vi "PH_Beckhoff_PP_Control.panel.vi"(0 "object ref":refnum<vi>, 5 "error in (no error)":errorcluster) -> (19 "error out":errorcluster)   [LabVIEW 2014, in "PH_Beckhoff_PP_Control.lvlib"]
doc: "This a GUI.\n\nLicense Agreement for this software:\n\nCopyright (C)\nGesellschaft für Schwerionenforschung, GSI\nPlanckstr. 1\n64291 Darmstadt\nGermany\n\nContact: D.Beck@gsi.de \n\nThis program is free software; you can redistribute it and/or modify it under the terms of the GNU General Public License as published by the Free Software Foundation; either version 2 of the license, or (at your option) any later version.\n\nThis program is distributed in the hope that it will be useful, but WITHOUT ANYW ARRANTY; without even the implied warranty of MERCHANTABILITY or FITNESS FOR A PARTICULAR PURPOSE. See the GNU General License for more details (http://www.gnu.org).\n\nGesellschaft für Schwerionenforschung, GSI\nPlanckstr. 1, 64291 Darmstadt, Germany\nFor all questions and ideas contact: M.Richter@gsi.de, H.Brand@gsi.de or D.Beck@gsi.de.\nLast update: 18-DEC-2002"
uses:
  PH_Beckhoff_PP_Control.lvlib
  PH_StatusHandler/PH_StatusHandler.GUI element.ctl
  PH_Beckhoff/PH_Beckhoff.Connectivity.ctl
  PH_Beckhoff/PH_Beckhoff.ADS Error.ctl
  PH_Beckhoff/PH_Beckhoff.Values.ctl
  PH_Beckhoff/PH_Beckhoff.Sonderklemmen Inputs.ctl
  PH_Beckhoff/PH_Beckhoff.Analog Inputs.ctl
  PH_Beckhoff/PH_Beckhoff.Scaling Type.ctl
  PH_Beckhoff/PH_Beckhoff.Analog Outputs.ctl
  PH_Beckhoff/PH_Beckhoff.Digital Inputs.ctl
  PH_Beckhoff/PH_Beckhoff.Digital Outputs.ctl
  PH_Beckhoff/PH_Beckhoff.GUI Refs.ctl
  CSCore/CSObj/CSObj.lvlib
  PH_Common/PH_Common.lvlib
  PH_Beckhoff/PH_Beckhoff.lvlib
  CSCore/CSSystem/CSSystemLib/CSSystemLib.lvlib
  PH_Class/PH_Class.lvlib
  PH_StatusHandler/PH_StatusHandler.lvlib
panel:
  in  "Tab Control":T1(tab)=enum."Mercury / Conductivity Control"
  out "Current Values":T2
  out "IP":string
  out "Connection":T9
  out "Prdc Int [ms]":i32
  out "ADS Error":T10
  out "configured?":bool
  in  "Show Info":bool
  out "Conductivity PSDB Status":u32(colorbox)=6618880 caption="PSDB"
  out "Mercury PSDB Status":u32(colorbox)=6618880 caption="PSDB"
  out "PP Conductivity Control":T12={"_Status"=0, "Device on"=16860, "Conductivity ok"=16860, "Temperature ok"=16860, "Alarm"=16860}
  out "PP Mercury Control":T13={"PHELIX Status"=0, "Device on"=16860, "Alarm"=16860, "on since:"="no info available", "Concentration"=0.0} caption="_Trigger 2 ..." {"Concentration" format="%#_7f"}
  in  "Delete":bool
  in  "Exit":bool
  # "PCS"
  # "3.40"
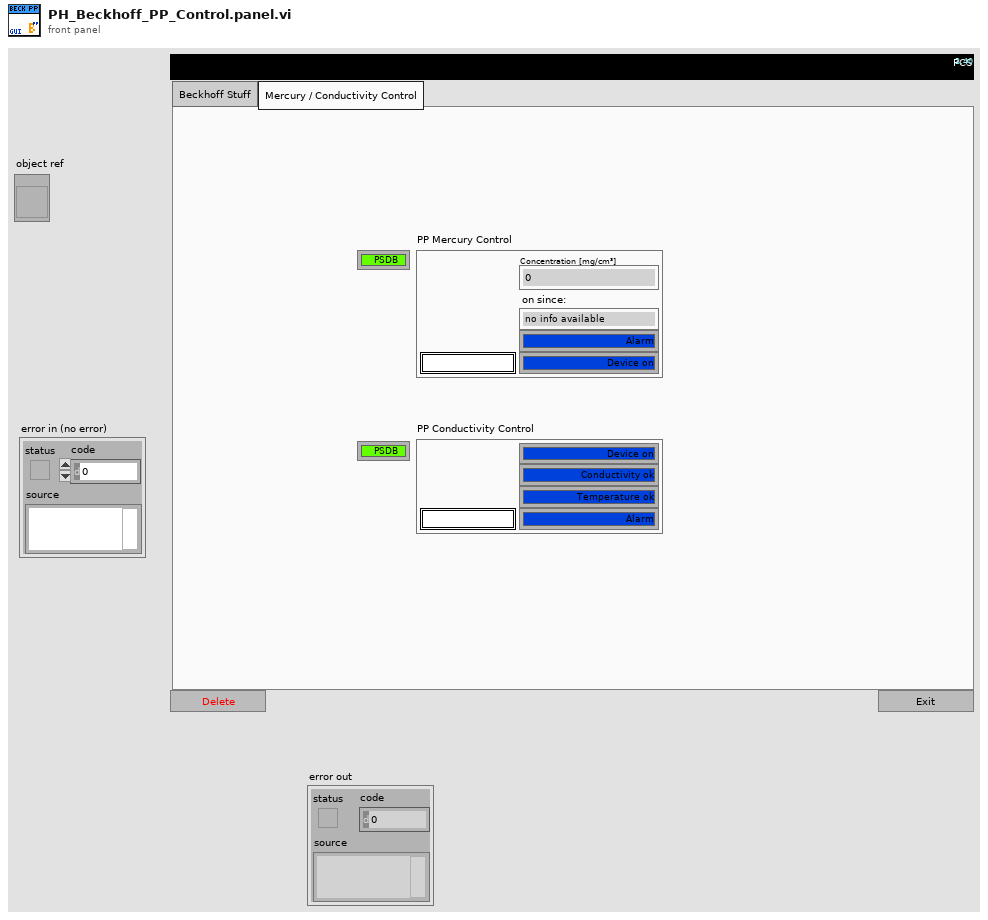
[diagram p1: front panel]
types:
  T1 = enum32{"Beckhoff Stuff", "Mercury / Conductivity Control"}
  T2 = typedef "PH_Beckhoff.lvlib/PH_Beckhoff.Values.ctl" = cluster{"Sonderklemmen Inputs":T3, "Analog Inputs":T4, "Analog Outputs":T6, "Digital Inputs":T7, "Digital Outputs":T8}
  T3 = typedef "PH_Beckhoff.lvlib/PH_Beckhoff.Sonderklemmen Inputs.ctl" = cluster{"Total Length":u32, "Name":string, "Value":u64, "Quality":bool, "Service ID":i32, "Offset":u32, "Length":u32}[]
  T4 = typedef "PH_Beckhoff.lvlib/PH_Beckhoff.Analog Inputs.ctl" = cluster{"Name":string, "Value":u32, "Quality":bool, "Service ID":i32, "Sca Type":T5}[]
  T5 = typedef "PH_Beckhoff.lvlib/PH_Beckhoff.Scaling Type.ctl" = enum16{"none", "0 ... 15 Bit -> 0 ... 5", "0 ... 15 Bit -> 0 ... 10", "0 ... 15 Bit -> 0 ... 25", "0 ... 15 Bit -> 4 ... 20", "0 ... 15 Bit -> 0 ... 1", "0 ... 15 Bit -> 0 ... 20000", "0 ... 15 Bit -> 0 ... 24000"}
  T6 = typedef "PH_Beckhoff.lvlib/PH_Beckhoff.Analog Outputs.ctl" = cluster{"Name":string, "Value":u32, "Quality":bool, "Wanted Value":u32, "Service ID":i32, "Sca Type":T5}[]
  T7 = typedef "PH_Beckhoff.lvlib/PH_Beckhoff.Digital Inputs.ctl" = cluster{"Name":string, "Value":bool, "Quality":bool, "Service ID":i32, "inverted?":bool}[]
  T8 = typedef "PH_Beckhoff.lvlib/PH_Beckhoff.Digital Outputs.ctl" = cluster{"Name":string, "Value":bool, "Quality":bool, "Wanted Value":bool, "Service ID":i32, "inverted?":bool}[]
  T9 = typedef "PH_Beckhoff.lvlib/PH_Beckhoff.Connectivity.ctl" = cluster{"DLL?":bool, "Port?":bool, "Client?":bool, "Ping?":bool, "unsuccessful Pings":u32}
  T10 = typedef "PH_Beckhoff.lvlib/PH_Beckhoff.ADS Error.ctl" = cluster{"Latest Error":string, "Error List":string[]}
  T11 = typedef "PH_StatusHandler.lvlib/PH_StatusHandler.GUI element.ctl" = u16
  T12 = cluster{"_Status":T11, "Device on":u32, "Conductivity ok":u32, "Temperature ok":u32, "Alarm":u32}
  T13 = cluster{"PHELIX Status":T11, "Device on":u32, "Alarm":u32, "on since:":string, "Concentration":dbl}
  T14 = typedef "PH_Beckhoff.lvlib/PH_Beckhoff.GUI Refs.ctl" = cluster{"ADS Error":refnum<vi>, "Values":refnum<vi>, "configured?":refnum<vi>, "Connection":refnum<vi>, "IP":refnum<vi>, "Prdc Int [ms]":refnum<vi>}
  T15 = typedef "PH_Beckhoff.lvlib/PH_Beckhoff.i attribute.ctl" = cluster{"GUI Refs":T14, "operation?":bool, "Default Prdc Interval":i32, "Connection":T9, "AMS Net ID":T16, "Klemmencluster: # of":T17, "Values":T2, "IP":string, "Description":string, "configured?":bool, "Change Manager":cluster{"Detemination wanted?":bool, "Values changed at":cluster{"Sonderklemmen Inputs":i32[], "Analog Inputs":i32[], "Analog Outputs":i32[], "Digital Inputs":i32[], "Digital Outputs":i32[]}}, "Difference to handle an analog input as change":u32}
  T16 = typedef "Beckhoff - Driver np.lvlib/Beckhoff Access.ctl" = cluster{"DLL path":path, "AMS Net ID":cluster{"1st # of IP":u8, "2nd # of IP":u8, "3rd # of IP":u8, "4th # of IP":u8, "In Port":u8, "Out Port":u8}}
  T17 = typedef "Beckhoff - Driver np.lvlib/Klemmendeclarer.ctl" = cluster{"Offset due to Sonderklemms":u32, "analog Inputs":u32, "analog Outputs":u32, "digital Input Bits":u32, "digital Output Bits":u32}
  T18 = typedef "PH_Beckhoff_PP_Control.lvlib/PH_Beckhoff_PP_Control.i attribute.ctl" = cluster{"PP Conductivity Control":cluster{"PSDB":cluster{"Status Service ID":i32, "Instance ID":i32, "Data Status":T19, "Ref Status":refnum<vi>, "Error Code":i32}, "Status":cluster{"GUI Ref":refnum<vi>, "Status Service ID":i32, "Status":T20}, "DIs":cluster{"Device on":cluster{"GUI Ref":refnum<vi>, "# in Data":i32}, "Conductivity ok":cluster{"GUI Ref":refnum<vi>, "# in Data":i32}, "Temperature ok":cluster{"GUI Ref":refnum<vi>, "# in Data":i32}, "Alarm":cluster{"GUI Ref":refnum<vi>, "# in Data":i32}}, "PSDB Thread":cluster{"Ref":refnum<vi>, "Q-Ref":refnum<queue>}}, "PP Mercury Control":cluster{"PSDB":cluster{"Status Service ID":i32, "Instance ID":i32, "Data Status":T19, "Ref Status":refnum<vi>, "Error Code":i32}, "Status":cluster{"GUI Ref":refnum<vi>, "Status Service ID":i32, "Status":T20}, "on since:":cluster{"GUI Ref":refnum<vi>, "Service ID":i32, "Time":string}, "DIs":cluster{"Device on":cluster{"GUI Ref":refnum<vi>, "# in Data":i32}, "Alarm":cluster{"GUI Ref":refnum<vi>, "# in Data":i32}}, "AIs":cluster{"Concentration":cluster{"GUI Ref":refnum<vi>, "# in Data":i32}}, "PSDB Thread":cluster{"Ref":refnum<vi>, "Q-Ref":refnum<queue>}}, "PSDB":cluster{"Shot #":i32, "Subsystem":T21}, "PSDB Credentials":T22}
  T19 = typedef "PH_PSDBWriter.lvlib/PH_PSDBWriter.Data Status.ctl" = i16
  T20 = typedef "PH_StatusHandler.lvlib/PH_StatusHandler.Status.ctl" = i16
  T21 = typedef "PH_PSDBWriter.lvlib/PH_PSDBWriter.PHELIX-Subsystems.ctl" = i32
  T22 = typedef "PH_Common.lvlib/PH_Connection.PSDB Credentials.ctl" = cluster{"PW":string, "ID":string, "DS":string}
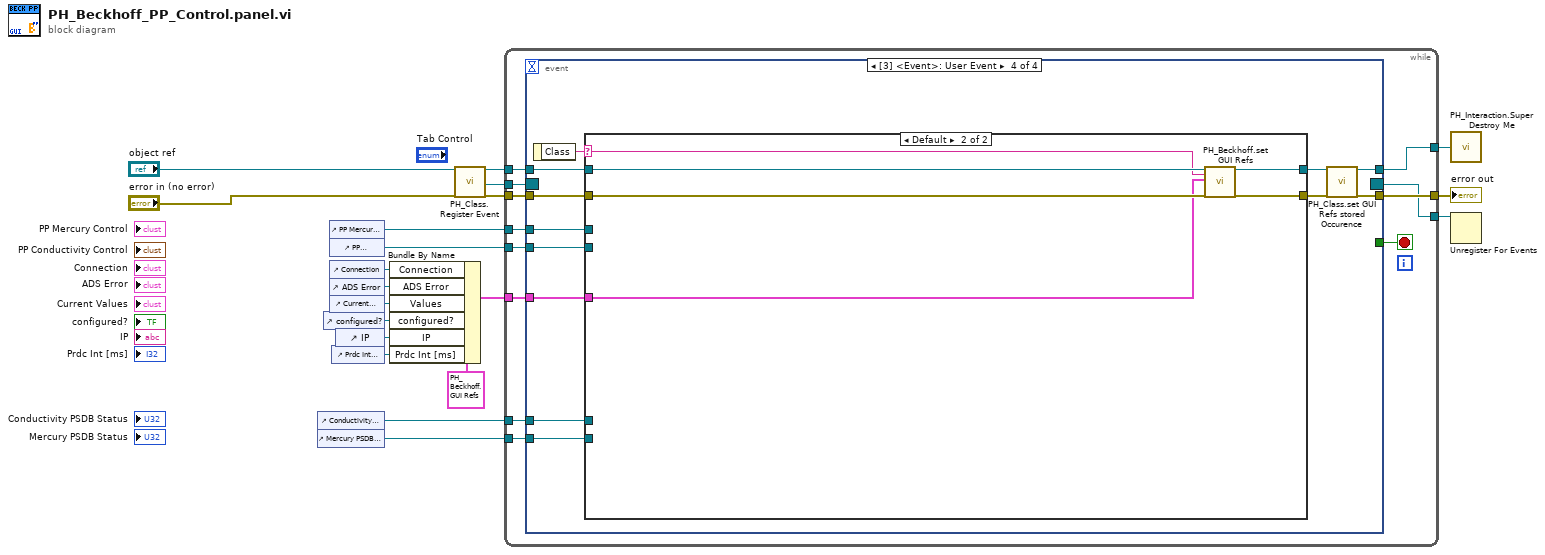
[diagram p0: block diagram]
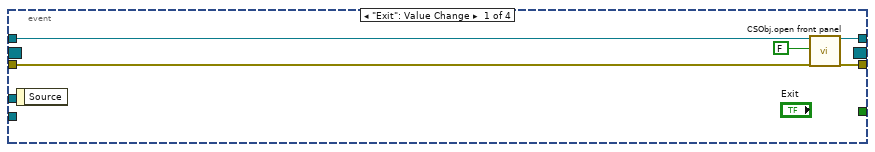
[diagram p2: hidden frame]
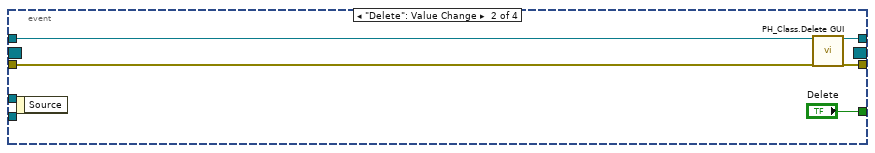
[diagram p3: hidden frame]
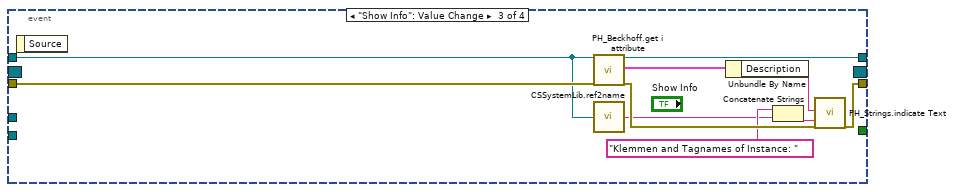
[diagram p4: hidden frame]
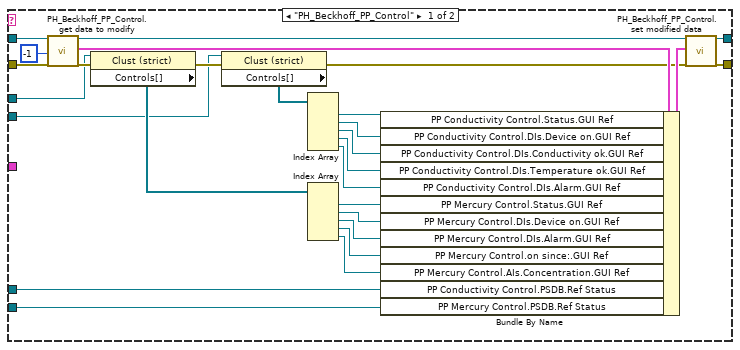
[diagram p5: hidden frame]
diagram:
  n1 = control-ref of="Conductivity PSDB Status"() -> (w6:refnum<vi>)
  n2 = control-ref of="Mercury PSDB Status"() -> (w5:refnum<vi>)
  n3 = control-ref of="configured?"() -> (w14:refnum<vi>)
  n4 = control-ref of="PP Mercury Control"() -> (w8:refnum<vi>)
  n5 = control-ref of="PP Conductivity Control"() -> (w7:refnum<vi>)
  n6 = control-ref of="Connection"() -> (w18:refnum<vi>)
  n7 = control-ref of="ADS Error"() -> (w17:refnum<vi>)
  n8 = control-ref of="Current Values"() -> (w15:refnum<vi>)
  n9 = control-ref of="Prdc Int [ms]"() -> (w1:refnum<vi>)
  n10 = control-ref of="IP"() -> (w2:refnum<vi>)
  n11 = Bundle By Name(cluster=T14 {"ADS Error"=refnum, "Values"=refnum, "configured?"=refnum, "Connection"=refnum, "IP"=refnum, "Prdc Int [ms]"=refnum} ("GUI Refs"), "Connection"=w18, "ADS Error"=w17, "Values"=w15, "configured?"=w14, "IP"=w2, "Prdc Int [ms]"=w1) -> (w9:T14)
  n12 = call "PH_Class.Register Event.vi"("i ref in"="object ref", "error in (no error)"="error in (no error)") -> ("i ref out"=w13:refnum<vi>, "Event Registration Refnum"=w11:refnum<event-registration>, "error out"=w12:errorcluster)  [unwired: 15 in]
  n13 = while {
    tunnel: w13 -> [w29]
    tunnel: [w28] -> w20
    tunnel: w12 -> [w31]
    tunnel: [w30] -> w19
    tunnel: w11 -> [w27]
    tunnel: [w26] -> w10
    tunnel: w9 -> [w25]
    tunnel: w8 -> [w24]
    tunnel: w7 -> [w23]
    tunnel: w6 -> [w22]
    tunnel: w5 -> [w21]
    stop <- w32 stop-if-true
    n14 = event shown="[3] <Event>: User Event" {
      selector: w27 -> [_ _ _ _]
      dyn-events: [_ _ _ _] -> w26
      timeout: _ -> [_ _ _ _]
      tunnel: [_ "Delete" _ _] -> w32
      tunnel: w29 -> [w34 w39 w43 w64]
      tunnel: w31 -> [w37 w41 w52 w63]
      tunnel: [w36 w40 w49 w55] -> w30
      tunnel: [w33 w38 w51 w53] -> w28
      tunnel: w25 -> [_ _ _ w61]
      tunnel: w24 -> [_ _ _ w59]
      tunnel: w23 -> [_ _ _ w58]
      tunnel: w22 -> [_ _ _ w57]
      tunnel: w21 -> [_ _ _ w56]
      event "Exit": Value Change {
        n15 = event-data() -> ()  [unwired: 1 in, 1 out]
        n16 = call "CSObj.open front panel.vi"("i ref in"=w34, "frontPanelOpen"=FALSE ("front panel open"), "error in (no error)"=w37) -> ("i ref out"=w33:refnum<vi>, "error out"=w36:errorcluster)  [unwired: 15 in]
      }
      event "Delete": Value Change {
        n17 = event-data() -> ()  [unwired: 1 in, 1 out]
        n18 = call "PH_Class.Delete GUI.vi"("VI in"=w39, "error in (no error)"=w41) -> ("VI out"=w38:refnum<vi>, "error out"=w40:errorcluster)  [unwired: 16 in]
      }
      event "Show Info": Value Change {
        n19 = event-data() -> ()  [unwired: 1 in, 1 out]
        n20 = call "PH_Beckhoff.get i attribute.vi"("i ref in"=w43, "error in (no error)"=w52) -> ("i ref out"=w51:refnum<vi>, "i attribute"=w48:T15, "error out"=w50:errorcluster)  [unwired: 15 in]
        n21 = call "CSSystemLib.ref2name.vi"("obj refnum"=w43) -> ("name"=w44:string)
        n22 = Unbundle By Name(w48) -> ("Description"=w47:string)
        n23 = Concatenate Strings("Klemmen and Tagnames of Instance: " ("Caption.Text"), w44) -> (w45:string)
        n24 = call "PH_Strings.indicate Text.vi"("String to show"=w47, "Caption.Text"=w45, "error in (no error)"=w50) -> ("error out"=w49:errorcluster)  [unwired: 16 in]
      }
      event User Event {
        n25 = event-data() -> ("Class"=w60:string)  [unwired: 1 in]
        n26 = case shown="Default" w60 {
          selector: w60 -> [_ w92]
          tunnel: w64 -> [w72 w97]
          tunnel: [w66 w96] -> w54
          tunnel: w63 -> [w71 w95]
          tunnel: [w65 w94] -> w62
          tunnel: w61 -> [_ w93]
          tunnel: w59 -> [w70 _]
          tunnel: w58 -> [w69 _]
          tunnel: w57 -> [w68 _]
          tunnel: w56 -> [w67 _]
          frame "PH_Beckhoff_PP_Control" {
            n27 = call "PH_Beckhoff_PP_Control.get data to modify.vi"("i ref in"=w72, "ms timeout (10000)"=-1, "error in (no error)"=w71) -> ("i ref out"=w91:refnum<vi>, "i attribute"=w90:T18, "error out"=w80:errorcluster)  [unwired: 13 in, 1 out]
            n28 = property class="Clust (strict)"(reference=w70, error in=w80) -> (error out=w79:errorcluster, "Controls[]"=w78:refnum<vi>[])  [unwired: 1 out]
            n29 = property class="Clust (strict)"(reference=w69, error in=w79) -> (error out=w86:errorcluster, "Controls[]"=w87:refnum<vi>[])  [unwired: 1 out]
            n30 = Index Array(array=w87) -> (element #1=w85:refnum<vi>, element #2=w84:refnum<vi>, element #3=w83:refnum<vi>, element #4=w82:refnum<vi>, element #5=w81:refnum<vi>)  [unwired: 5 in]
            n31 = Index Array(array=w78) -> (element #1=w77:refnum<vi>, element #2=w76:refnum<vi>, element #3=w75:refnum<vi>, element #4=w74:refnum<vi>, element #5=w73:refnum<vi>)  [unwired: 5 in]
            n32 = Bundle By Name(cluster=w90, "PP Conductivity Control.Status.GUI Ref"=w85, "PP Conductivity Control.DIs.Device on.GUI Ref"=w84, "PP Conductivity Control.DIs.Conductivity ok.GUI Ref"=w83, "PP Conductivity Control.DIs.Temperature ok.GUI Ref"=w82, "PP Conductivity Control.DIs.Alarm.GUI Ref"=w81, "PP Mercury Control.Status.GUI Ref"=w77, "PP Mercury Control.DIs.Device on.GUI Ref"=w76, "PP Mercury Control.DIs.Alarm.GUI Ref"=w75, "PP Mercury Control.on since:.GUI Ref"=w74, "PP Mercury Control.AIs.Concentration.GUI Ref"=w73, "PP Conductivity Control.PSDB.Ref Status"=w68, "PP Mercury Control.PSDB.Ref Status"=w67) -> (w88:T18)
            n33 = call "PH_Beckhoff_PP_Control.set modified data.vi"("i ref in"=w91, "i attribute"=w88, "error in (no error)"=w86) -> ("i ref out"=w66:refnum<vi>, "error out"=w65:errorcluster)  [unwired: 15 in]
          }
          frame Default {
            n34 = call "PH_Beckhoff.set GUI Refs.vi"("i ref in"=w97, "Class"=w92, "GUI Refs"=w93, "error in"=w95) -> ("i ref out"=w96:refnum<vi>, "error out"=w94:errorcluster)  [unwired: 14 in]
          }
        }
        n35 = call "PH_Class.set GUI Refs stored Occurence.vi"("i ref in"=w54, "error in (no error)"=w62) -> ("i ref out"=w53:refnum<vi>, "error out"=w55:errorcluster)  [unwired: 16 in]
      }
    }
  }
  "error out" <- w19
  n36 = call "PH_Interaction.Super Destroy Me.vi"("i ref out"=w20) -> ()
  n37 = Unregister For Events(event registration refnum=w10) -> ()  [unwired: 1 in, 1 out]
